vi "保存参数.vi"(0 "设置文件路径":path, 1 "设置":T1, 3 "error in (no error)":errorcluster caption="错误输入（无错误）") -> (9 "error out":errorcluster caption="错误输出")   [LabVIEW 2018]
uses:
  <vilib>/Utility/config.llb/Write Key (U32).vi
  <vilib>/Utility/config.llb/Write Key (String).vi
  <vilib>/Utility/config.llb/Write Key (Double).vi
  <vilib>/Utility/config.llb/Write Key (I32).vi
  <vilib>/Utility/config.llb/NI_LVConfig.lvlib
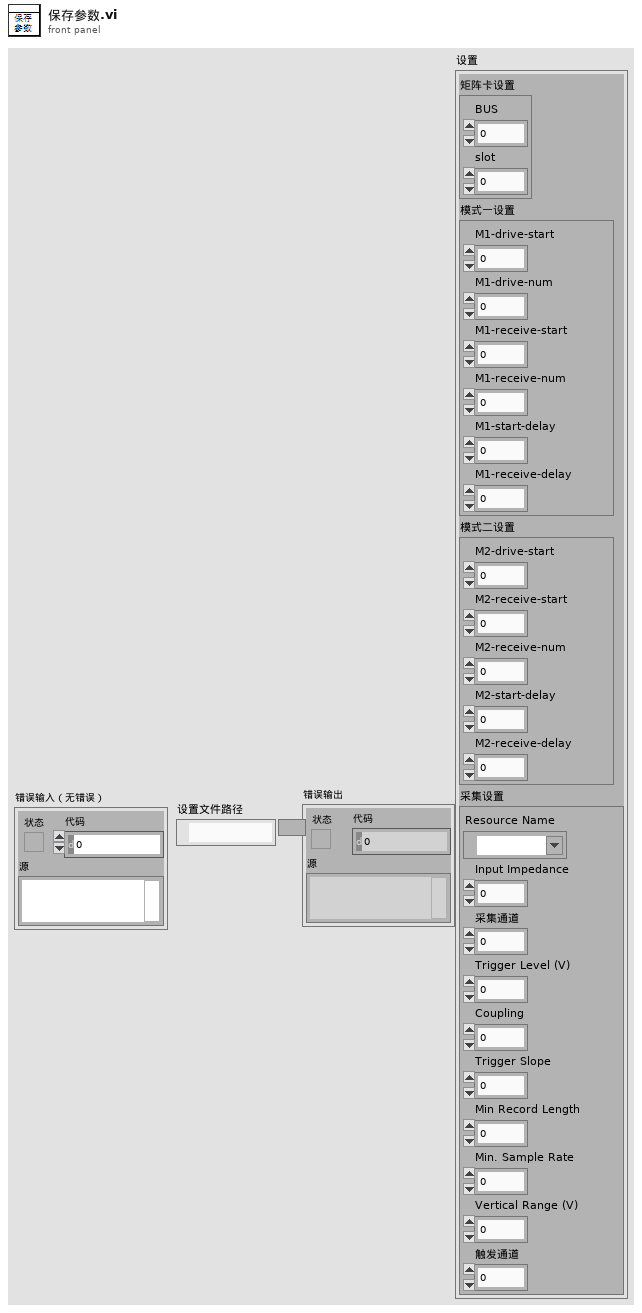
[diagram p1: front panel]
types:
  T1 = cluster{"矩阵卡设置":cluster{"BUS":u32, "slot":u32}, "模式一设置":cluster{"M1-drive-start":u32, "M1-drive-num":u32, "M1-receive-start":u32, "M1-receive-num":u32, "M1-start-delay":u32, "M1-receive-delay":u32}, "模式二设置":cluster{"M2-drive-start":u32, "M2-receive-start":u32, "M2-receive-num":u32, "M2-start-delay":u32, "M2-receive-delay":u32}, "采集设置":cluster{"Resource Name":refnum<k15>, "Input Impedance":u32, "采集通道":i32, "Trigger Level (V)":dbl, "Coupling":u16, "Trigger Slope":i32, "Min Record Length":i32, "Min. Sample Rate":dbl, "Vertical Range (V)":dbl, "触发通道":i32}}
  T2 = typedef "NI_LVConfig.lvlib/Config Data RefNum.ctl" = refnum<k1>
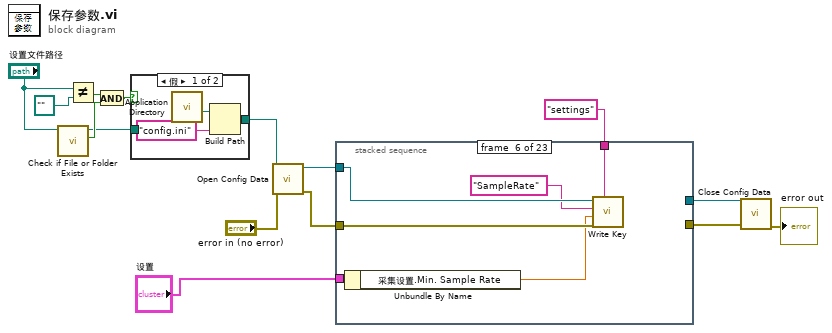
[diagram p0: block diagram]
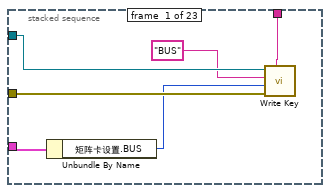
[diagram p3: hidden frame]
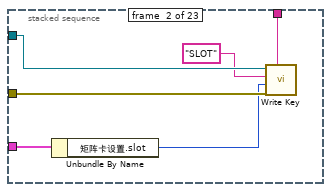
[diagram p4: hidden frame]
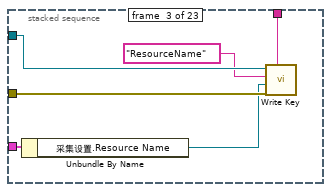
[diagram p5: hidden frame]
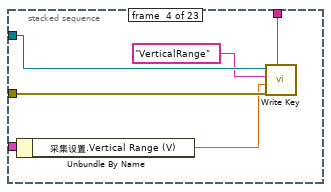
[diagram p6: hidden frame]
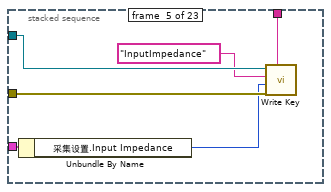
[diagram p7: hidden frame]
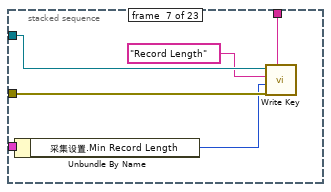
[diagram p8: hidden frame]
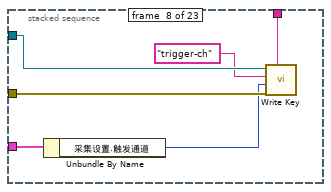
[diagram p9: hidden frame]
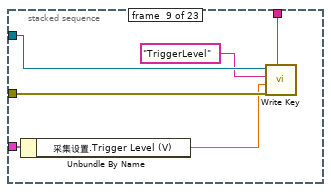
[diagram p10: hidden frame]
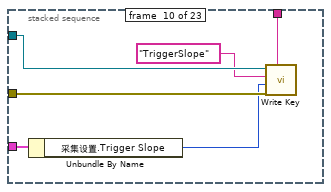
[diagram p11: hidden frame]
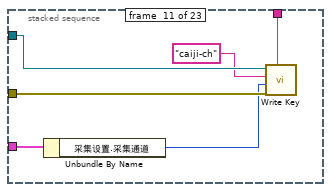
[diagram p12: hidden frame]
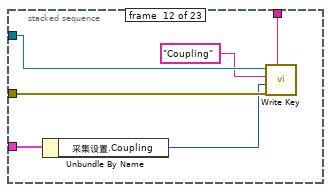
[diagram p13: hidden frame]
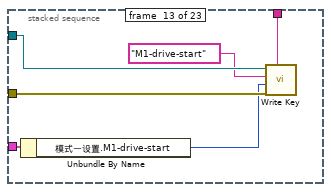
[diagram p14: hidden frame]
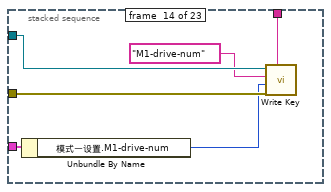
[diagram p15: hidden frame]
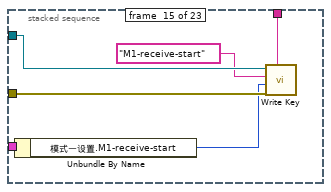
[diagram p16: hidden frame]
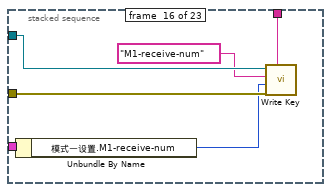
[diagram p17: hidden frame]
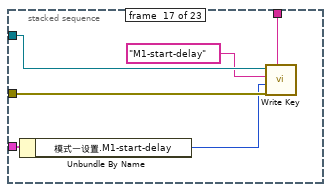
[diagram p18: hidden frame]
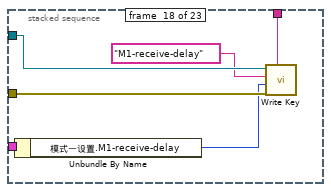
[diagram p19: hidden frame]
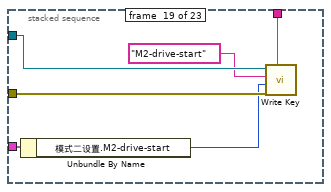
[diagram p20: hidden frame]
diagram:
  n1 = call <vilib>:"Check if File or Folder Exists.vi"("path"="设置文件路径") -> ("file or folder exists?"=w5:bool, "dup path"=w3:path)  [unwired: 8 in, 1 out]
  n2 = Not Equal?(x="设置文件路径", y=path "" ("添加的路径")) -> (x != y?=w6:bool)
  n3 = And(x=w6, y=w5) -> (x .and. y?=w4:bool)
  n4 = case shown="假" w4 {
    tunnel: [w16 w19] -> w2
    tunnel: w3 -> [_ w19]
    frame False {
      n5 = call <vilib>:"Application Directory.vi"() -> ("Application Directory"=w18:path)
      n6 = Build Path(base path=w18, name or relative path="config.ini" ("名称或相对路径")) -> (appended path=w16:path)
    }
    frame True {
    }
  }
  n7 = call <vilib>:"Open Config Data.vi"("error in (no error)"="error in (no error)", "configuration file path"=w2) -> ("error out"=w14:errorcluster, "refnum"=w15:T2)  [unwired: 7 in, 1 out]
  n8 = stacked-sequence {
    tunnel: w15 -> [w23 w30 w36 w42 w48 w54 w60 w66 w72 w78 w84 w90 w96 w102 w108 w114 w120 w126 w132 w138 w144 w150 w158]
    tunnel: w14 -> [w24 w29 w35 w41 w47 w53 w59 w65 w71 w77 w83 w89 w95 w101 w107 w113 w119 w125 w131 w137 w143 w149 w157]
    tunnel: "settings" ("section") -> [w25 w31 w37 w43 w49 w55 w61 w67 w73 w79 w85 w91 w97 w103 w109 w115 w121 w127 w133 w139 w145 w151 w159]
    tunnel: "设置" -> [w22 w28 w34 w40 w46 w52 w58 w64 w70 w76 w82 w88 w94 w100 w106 w112 w118 w124 w130 w136 w142 w148 w156]
    tunnel: [_ _ _ _ _ _ _ _ _ _ _ _ _ _ _ _ _ _ _ _ _ _ w153] -> w12
    tunnel: [_ _ _ _ _ _ _ _ _ _ _ _ _ _ _ _ _ _ _ _ _ _ w152] -> w11
    frame #0 {
      n9 = Unbundle By Name(w22) -> ("矩阵卡设置.BUS"=w20:u32)
      n10 = call-poly <vilib>:"Write Key.vi"("section"=w25, "error in (no error)"=w24, "value"=w20, "key"="BUS", "refnum"=w23) -> ()  [unwired: 4 in, 3 out]
    }
    frame #1 {
      n11 = Unbundle By Name(w28) -> ("矩阵卡设置.slot"=w26:u32)
      n12 = call-poly <vilib>:"Write Key.vi"("section"=w31, "error in (no error)"=w29, "value"=w26, "key"="SLOT", "refnum"=w30) -> ()  [unwired: 4 in, 3 out]
    }
    frame #2 {
      n13 = Unbundle By Name(w34) -> ("采集设置.Resource Name"=w32:refnum<k15>)
      n14 = call-poly <vilib>:"Write Key.vi"("section"=w37, "error in (no error)"=w35, "value"=w32, "key"="ResourceName", "refnum"=w36) -> ()  [unwired: 4 in, 3 out]
    }
    frame #3 {
      n15 = Unbundle By Name(w40) -> ("采集设置.Vertical Range (V)"=w38:dbl)
      n16 = call-poly <vilib>:"Write Key.vi"("section"=w43, "error in (no error)"=w41, "value"=w38, "key"="VerticalRange", "refnum"=w42) -> ()  [unwired: 4 in, 3 out]
    }
    frame #4 {
      n17 = Unbundle By Name(w46) -> ("采集设置.Input Impedance"=w44:u32)
      n18 = call-poly <vilib>:"Write Key.vi"("section"=w49, "error in (no error)"=w47, "value"=w44, "key"="InputImpedance", "refnum"=w48) -> ()  [unwired: 4 in, 3 out]
    }
    frame #5 {
      n19 = Unbundle By Name(w52) -> ("采集设置.Min. Sample Rate"=w50:dbl)
      n20 = call-poly <vilib>:"Write Key.vi"("section"=w55, "error in (no error)"=w53, "value"=w50, "key"="SampleRate", "refnum"=w54) -> ()  [unwired: 4 in, 3 out]
    }
    frame #6 {
      n21 = Unbundle By Name(w58) -> ("采集设置.Min Record Length"=w56:i32)
      n22 = call-poly <vilib>:"Write Key.vi"("section"=w61, "error in (no error)"=w59, "value"=w56, "key"="Record Length", "refnum"=w60) -> ()  [unwired: 4 in, 3 out]
    }
    frame #7 {
      n23 = Unbundle By Name(w64) -> ("采集设置.触发通道"=w62:i32)
      n24 = call-poly <vilib>:"Write Key.vi"("section"=w67, "error in (no error)"=w65, "value"=w62, "key"="trigger-ch", "refnum"=w66) -> ()  [unwired: 4 in, 3 out]
    }
    frame #8 {
      n25 = Unbundle By Name(w70) -> ("采集设置.Trigger Level (V)"=w68:dbl)
      n26 = call-poly <vilib>:"Write Key.vi"("section"=w73, "error in (no error)"=w71, "value"=w68, "key"="TriggerLevel", "refnum"=w72) -> ()  [unwired: 4 in, 3 out]
    }
    frame #9 {
      n27 = Unbundle By Name(w76) -> ("采集设置.Trigger Slope"=w74:i32)
      n28 = call-poly <vilib>:"Write Key.vi"("section"=w79, "error in (no error)"=w77, "value"=w74, "key"="TriggerSlope", "refnum"=w78) -> ()  [unwired: 4 in, 3 out]
    }
    frame #10 {
      n29 = Unbundle By Name(w82) -> ("采集设置.采集通道"=w80:i32)
      n30 = call-poly <vilib>:"Write Key.vi"("section"=w85, "error in (no error)"=w83, "value"=w80, "key"="caiji-ch", "refnum"=w84) -> ()  [unwired: 4 in, 3 out]
    }
    frame #11 {
      n31 = Unbundle By Name(w88) -> ("采集设置.Coupling"=w86:u16)
      n32 = call-poly <vilib>:"Write Key.vi"("section"=w91, "error in (no error)"=w89, "value"=w86, "key"="Coupling", "refnum"=w90) -> ()  [unwired: 4 in, 3 out]
    }
    frame #12 {
      n33 = Unbundle By Name(w94) -> ("模式一设置.M1-drive-start"=w92:u32)
      n34 = call-poly <vilib>:"Write Key.vi"("section"=w97, "error in (no error)"=w95, "value"=w92, "key"="M1-drive-start", "refnum"=w96) -> ()  [unwired: 4 in, 3 out]
    }
    frame #13 {
      n35 = Unbundle By Name(w100) -> ("模式一设置.M1-drive-num"=w98:u32)
      n36 = call-poly <vilib>:"Write Key.vi"("section"=w103, "error in (no error)"=w101, "value"=w98, "key"="M1-drive-num", "refnum"=w102) -> ()  [unwired: 4 in, 3 out]
    }
    frame #14 {
      n37 = Unbundle By Name(w106) -> ("模式一设置.M1-receive-start"=w104:u32)
      n38 = call-poly <vilib>:"Write Key.vi"("section"=w109, "error in (no error)"=w107, "value"=w104, "key"="M1-receive-start", "refnum"=w108) -> ()  [unwired: 4 in, 3 out]
    }
    frame #15 {
      n39 = Unbundle By Name(w112) -> ("模式一设置.M1-receive-num"=w110:u32)
      n40 = call-poly <vilib>:"Write Key.vi"("section"=w115, "error in (no error)"=w113, "value"=w110, "key"="M1-receive-num", "refnum"=w114) -> ()  [unwired: 4 in, 3 out]
    }
    frame #16 {
      n41 = Unbundle By Name(w118) -> ("模式一设置.M1-start-delay"=w116:u32)
      n42 = call-poly <vilib>:"Write Key.vi"("section"=w121, "error in (no error)"=w119, "value"=w116, "key"="M1-start-delay", "refnum"=w120) -> ()  [unwired: 4 in, 3 out]
    }
    frame #17 {
      n43 = Unbundle By Name(w124) -> ("模式一设置.M1-receive-delay"=w122:u32)
      n44 = call-poly <vilib>:"Write Key.vi"("section"=w127, "error in (no error)"=w125, "value"=w122, "key"="M1-receive-delay", "refnum"=w126) -> ()  [unwired: 4 in, 3 out]
    }
    frame #18 {
      n45 = Unbundle By Name(w130) -> ("模式二设置.M2-drive-start"=w128:u32)
      n46 = call-poly <vilib>:"Write Key.vi"("section"=w133, "error in (no error)"=w131, "value"=w128, "key"="M2-drive-start", "refnum"=w132) -> ()  [unwired: 4 in, 3 out]
    }
    frame #19 {
      n47 = Unbundle By Name(w136) -> ("模式二设置.M2-receive-start"=w134:u32)
      n48 = call-poly <vilib>:"Write Key.vi"("section"=w139, "error in (no error)"=w137, "value"=w134, "key"="M2-receive-start", "refnum"=w138) -> ()  [unwired: 4 in, 3 out]
    }
    frame #20 {
      n49 = Unbundle By Name(w142) -> ("模式二设置.M2-receive-num"=w140:u32)
      n50 = call-poly <vilib>:"Write Key.vi"("section"=w145, "error in (no error)"=w143, "value"=w140, "key"="M2-receive-num", "refnum"=w144) -> ()  [unwired: 4 in, 3 out]
    }
    frame #21 {
      n51 = Unbundle By Name(w148) -> ("模式二设置.M2-start-delay"=w146:u32)
      n52 = call-poly <vilib>:"Write Key.vi"("section"=w151, "error in (no error)"=w149, "value"=w146, "key"="M2-start-delay", "refnum"=w150) -> ()  [unwired: 4 in, 3 out]
    }
    frame #22 {
      n53 = Unbundle By Name(w156) -> ("模式二设置.M2-receive-delay"=w154:u32)
      n54 = call-poly <vilib>:"Write Key.vi"("section"=w159, "error in (no error)"=w157, "value"=w154, "key"="M2-receive-delay", "refnum"=w158) -> ("error out"=w152:errorcluster, "refnum out"=w153:T2)  [unwired: 4 in, 1 out]
    }
  }
  n55 = call <vilib>:"Close Config Data.vi"("error in (no error)"=w11, "refnum"=w12) -> ("error out"=→"error out":errorcluster)  [unwired: 8 in, 1 out]
